vi "DSF.Engine.Thread Parameters.Create.vi"(8 "error in (no error)":errorcluster, 9 "id":i32, 10 "processor":i32=-2, 11 "priority":i32=100) -> (0 "error out":errorcluster, 3 "Thread Parameters":refnum<class "Thread Parameters.lvclass">)   [LabVIEW 2017, in "Data Sharing Framework Engine.lvlib" / "Thread Parameters.lvclass"]
uses:
  Thread Parameters.lvclass
  Thread Parameters.lvclass/Thread Parameters.ctl
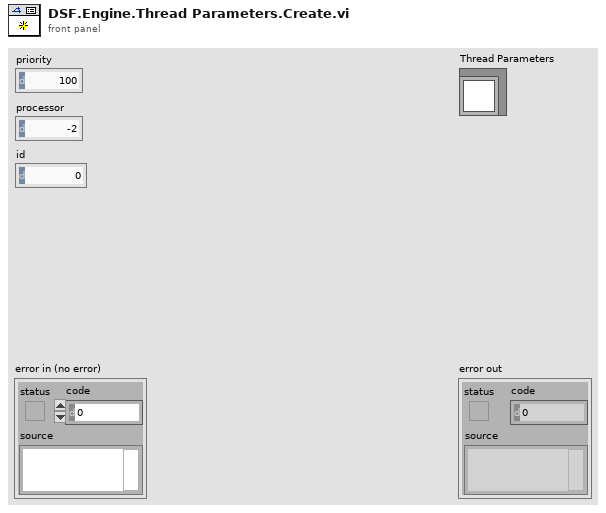
[diagram p1: front panel]
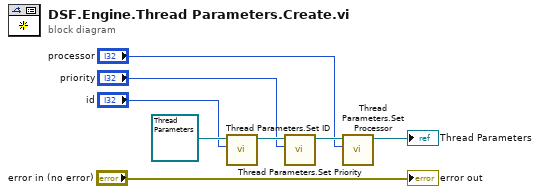
[diagram p0: block diagram]
diagram:
  n1 = call "Thread Parameters.Set ID.vi"("id"="id", "Plugin in"=refnum<class "Thread Parameters.lvclass"> refnum ("Thread Parameters in")) -> ("Plugin out"=w7:refnum<class "Thread Parameters.lvclass">)  [unwired: 9 in]
  n2 = call "Thread Parameters.Set Priority.vi"("Priority"="priority", "Thread Parameters in"=w7) -> ("Thread Parameters out"=w6:refnum<class "Thread Parameters.lvclass">)  [unwired: 9 in]
  n3 = call "Thread Parameters.Set Processor.vi"("Processor"="processor", "Thread Parameters in"=w6) -> ("Thread Parameters out"=→"Thread Parameters":refnum<class "Thread Parameters.lvclass">)  [unwired: 9 in]
  "error out" <- "error in (no error)"
